vi "Save Config File.vi"(8 "error in":errorcluster, 10 "text":string, 11 "base path":path) -> (0 "error out":errorcluster)   [LabVIEW 2017]
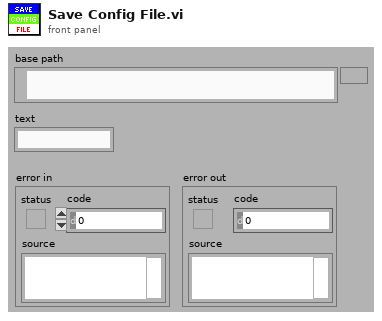
[diagram p1: front panel]
types:
  T1 = enum16{"open", "replace", "create", "open or create", "replace or create", "replace or create with confirmation"}
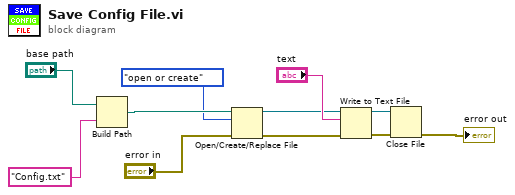
[diagram p0: block diagram]
diagram:
  n1 = Build Path(base path="base path", name or relative path="Config.txt") -> (appended path=w9:path)
  n2 = Open/Create/Replace File(file path (use dialog)=w9, error in="error in", operation (0:open)=T1."open or create") -> (refnum out=w1:refnum<file>, error out=w2:errorcluster)  [unwired: 4 out]
  n3 = Write to Text File(file (use dialog)=w1, text="text", error in=w2) -> (refnum out=w11:refnum<file>, error out=w10:errorcluster)  [unwired: 1 in, 1 out]
  n4 = Close File(refnum=w11, error in=w10) -> (error out=→"error out":errorcluster)  [unwired: 1 out]
